vi "ConnectToRobot.vi"(0 "error in":errorcluster, 1 "ip":string, 3 "Enable Dashboard":bool, 4 "Enable Primary Interface":bool, 5 "RTDE Connect Parameters":refnum<k24>) -> (14 "error out":errorcluster, 15 "UR Robot":refnum<k24>, 17 "Dashboard":refnum<k24>, 18 "PrimaryInterface":refnum<k24>, 19 "Rtde":refnum<k24>)   [LabVIEW 2023, in "UnderAutomation.UniversalRobots.lvlib"]
uses:
  UnderAutomation.UniversalRobots.lvlib
  C:/Users/fg/Documents/UniversalRobots.vi/UnderAutomation.UniversalRobots/lib/UnderAutomation.UniversalRobots.dll
  lib/UnderAutomation.UniversalRobots.dll
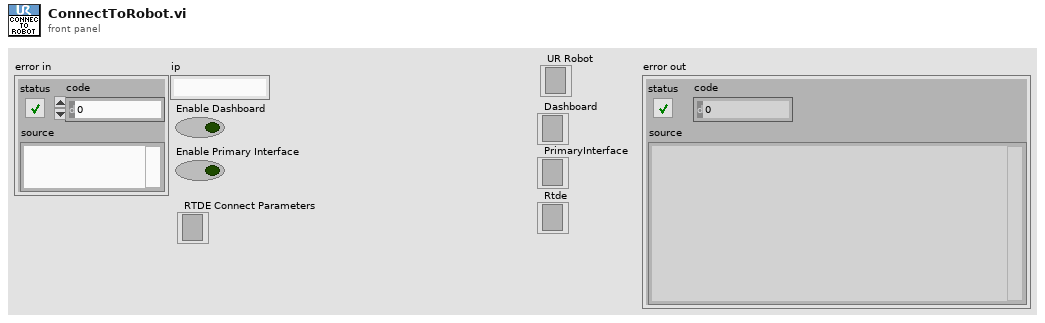
[diagram p1: front panel]
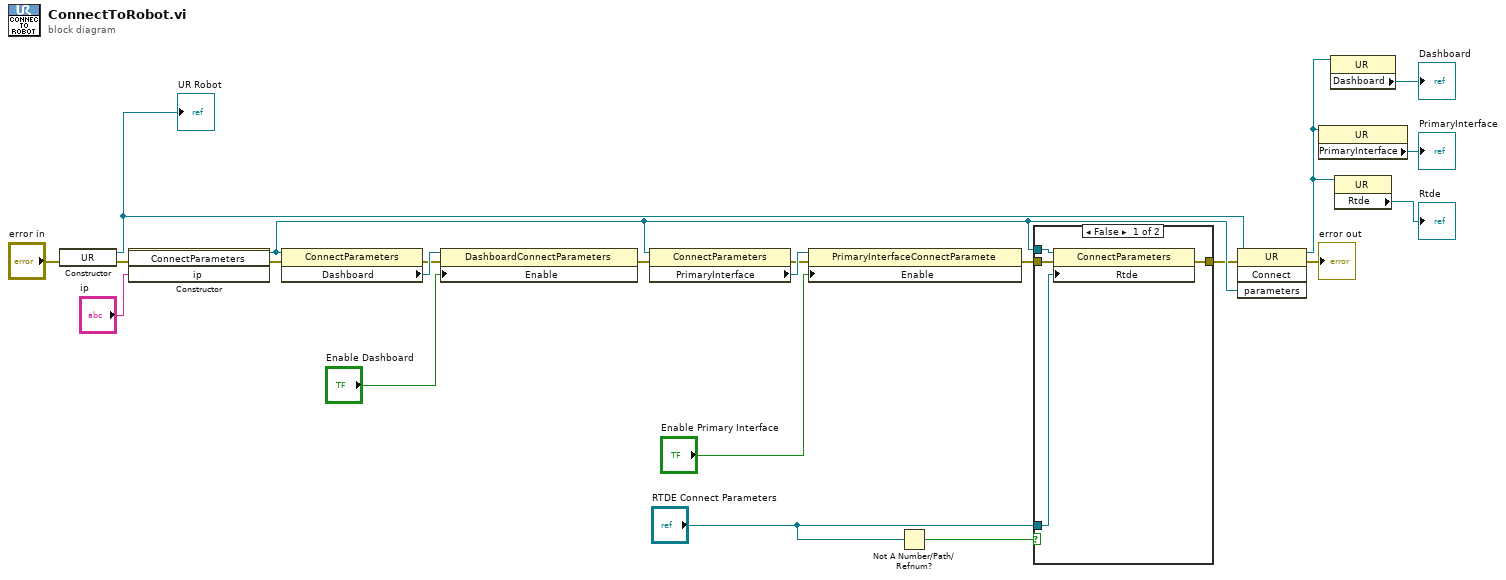
[diagram p0: block diagram]
diagram:
  n1 = constructor class="UR"(error in="error in") -> (reference out=w1:refnum<k24>, error out=w18:errorcluster)  [unwired: 2 in, 1 out]
  "UR Robot" <- w1
  n2 = constructor class="ConnectParameters"(error in=w18, "ip"="ip") -> (reference out=w9:refnum<k24>, error out=w17:errorcluster)  [unwired: 2 in, 2 out]
  n3 = property class="ConnectParameters"(reference=w9, error in=w17) -> (error out=w16:errorcluster, "Dashboard"=w20:refnum<k24>)  [unwired: 1 out]
  n4 = property class="DashboardConnectParameters"(reference=w20, error in=w16, "Enable"="Enable Dashboard") -> (error out=w15:errorcluster)  [unwired: 1 out]
  n5 = property class="ConnectParameters"(reference=w9, error in=w15) -> (error out=w14:errorcluster, "PrimaryInterface"=w19:refnum<k24>)  [unwired: 1 out]
  n6 = property class="PrimaryInterfaceConnectParamete"(reference=w19, error in=w14, "Enable"="Enable Primary Interface") -> (error out=w7:errorcluster)  [unwired: 1 out]
  n7 = Not A Number/Path/Refnum?(number/path/refnum="RTDE Connect Parameters") -> (NaN/Path/Refnum?=w10:bool)
  n8 = case shown="False" w10 {
    tunnel: w9 -> [w26 _]
    tunnel: "RTDE Connect Parameters" -> [w25 _]
    tunnel: w7 -> [w24 w27]
    tunnel: [w23 w27] -> w6
    frame False {
      n9 = property class="ConnectParameters"(reference=w26, error in=w24, "Rtde"=w25) -> (error out=w23:errorcluster)  [unwired: 1 out]
    }
    frame True {
    }
  }
  n10 = invoke class="UR" method="Connect"(reference=w1, error in=w6, "parameters"=w9) -> (reference out=w3:refnum<k24>, error out=→"error out":errorcluster)  [unwired: 1 in, 2 out]
  n11 = property class="UR"(reference=w3) -> ("PrimaryInterface"=→"PrimaryInterface":refnum<k24>)  [unwired: 1 in, 2 out]
  n12 = property class="UR"(reference=w3) -> ("Dashboard"=→"Dashboard":refnum<k24>)  [unwired: 1 in, 2 out]
  n13 = property class="UR"(reference=w3) -> ("Rtde"=→"Rtde":refnum<k24>)  [unwired: 1 in, 2 out]
